vi "send_SteeringControl.vi"(4 "Counter":i32, 5 "200/freq":i32=20, 6 "Active":bool, 7 "CAN ID":u32=656 format="%x", 8 "Message":T1={"Rot. sw 4"=1, "Rot. sw 5"=1, "Rot. sw 3"=1, "Rot. sw 1"=1, "Rot. sw 2"=1, "Button 3"=FALSE, "Button 1"=FALSE, "Button 2"=FALSE, "Button 4"=FALSE} {"Rot. sw 2" min=1 max=12 scale=1.0..12.0; "Rot. sw 1" min=1 max=12 scale=1.0..12.0; "Rot. sw 3" min=1 max=12 scale=1.0..12.0; "Rot. sw 5" min=1 max=12 scale=1.0..12.0; "Rot. sw 4" min=1 max=12 scale=1.0..12.0}, 11 "CAN frame":T2[](array[typedef]) {"Data" format="%.0x"; "ArbitrationId" format="%.0x"; "Timestamp" format="%<%I:%M:%S%3u %p\n%m/%d/%Y>T"}) -> (3 "CAN frame out":T2[](array[typedef]) {"Data" format="%.0x"; "ArbitrationId" format="%.0x"; "Timestamp" format="%<%I:%M:%S%3u %p\n%m/%d/%Y>T"})   [LabVIEW 2017]
uses:
  <vilib>/nican/nican.llb/CanFrameTimed.ctl
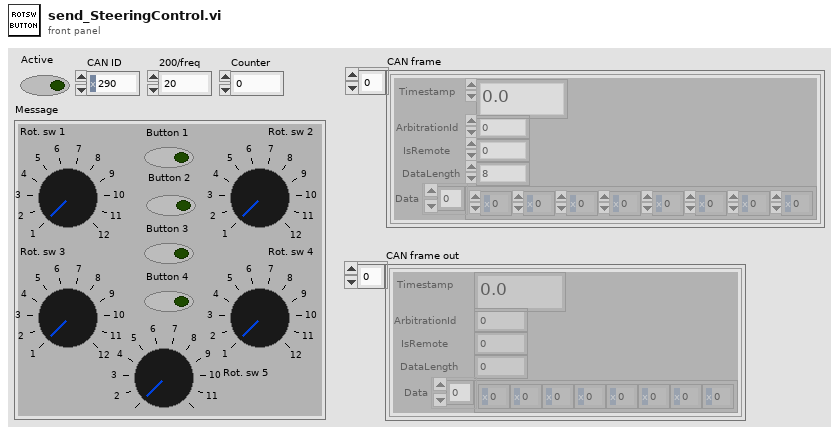
[diagram p1: front panel]
types:
  T1 = cluster{"Rot. sw 4":u16, "Rot. sw 5":u16, "Rot. sw 3":u16, "Rot. sw 1":u16, "Rot. sw 2":u16, "Button 3":bool, "Button 1":bool, "Button 2":bool, "Button 4":bool}
  T2 = typedef "CanFrameTimed.ctl" = cluster{"Timestamp":dbl, "ArbitrationId":u32, "IsRemote":u8, "DataLength":u8, "Data":u8[]}
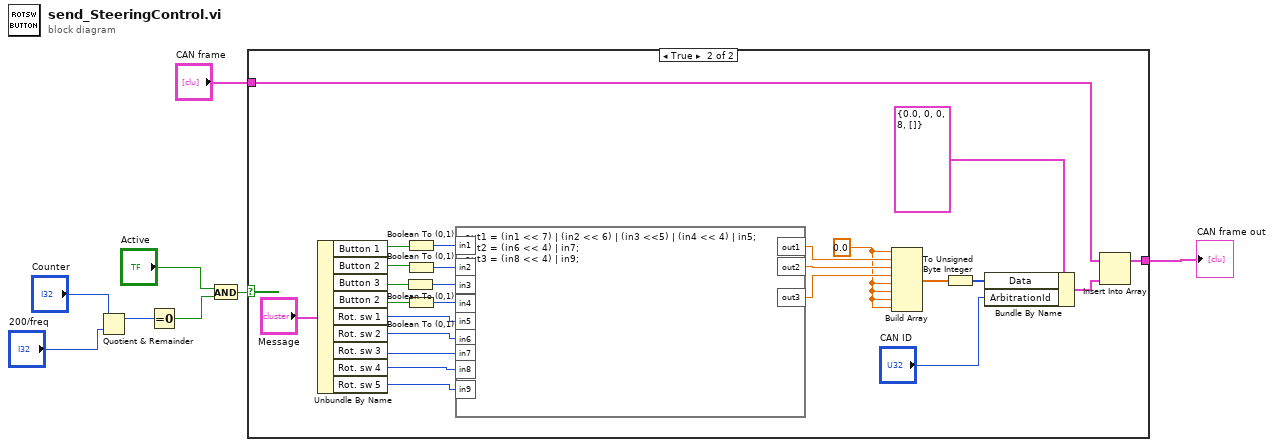
[diagram p0: block diagram]
diagram:
  n1 = Quotient & Remainder(x="Counter", y="200/freq") -> (x-y*floor(x/y)=w5:i32)  [unwired: 1 out]
  n2 = Equal To 0?(x=w5) -> (x = 0?=w3:bool)
  n3 = And(x="Active", y=w3) -> (x .and. y?=w2:bool)
  n4 = case shown="True" w2 {
    tunnel: "CAN frame" -> [w9 w31]
    tunnel: [w9 w29] -> w7
    frame False {
    }
    frame True {
      w11 = 0.0 ("element")
      n5 = Unbundle By Name("Message") -> ("Button 1"=w20:bool, "Button 2"=w19:bool, "Button 3"=w21:bool, "Button 2"=w23:bool, "Rot. sw 1"=w24:u16, "Rot. sw 2"=w25:u16, "Rot. sw 3"=w26:u16, "Rot. sw 4"=w27:u16, "Rot. sw 5"=w28:u16)
      n6 = Boolean To (0,1)(Boolean=w21) -> (0, 1=w16:i16)
      n7 = Boolean To (0,1)(Boolean=w20) -> (0, 1=w15:i16)
      n8 = Boolean To (0,1)(Boolean=w19) -> (0, 1=w18:i16)
      n9 = Boolean To (0,1)(Boolean=w23) -> (0, 1=w22:i16)
      n10 = formula code="out1 = (in1 << 7) | (in2 << 6) | (in3 <<5) | (in4 << 4) | in5;\nout2 = (in6 << 4) | in7;\nout3 = (in8 << 4) | in9;"("in1"=w15, "in2"=w18, "in3"=w16, "in4"=w22, "in5"=w24, "in6"=w25, "in7"=w26, "in8"=w27, "in9"=w28) -> ("out1"=w14:dbl, "out2"=w13:dbl, "out3"=w12:dbl)
      n11 = Build Array(w11, w14, w13, w12, w11, w11, w11, w11) -> (w34:dbl[])
      n12 = To Unsigned Byte Integer(number=w34) -> (unsigned 8bit integer=w33:u8[])
      n13 = Bundle By Name(cluster=T2 {"Timestamp"=0.0, "ArbitrationId"=0, "IsRemote"=0, "DataLength"=8, "Data"=[]} ("CAN frame"), "Data"=w33, "ArbitrationId"="CAN ID") -> (w30:T2)
      n14 = Insert Into Array(array=w31, new element=w30) -> (w29:T2[])  [unwired: 1 in]
    }
  }
  "CAN frame out" <- w7
